vi "onListenForNewConnection.vi"(8 "error in (no error)":errorcluster, 9 "timeout (ms)":i32=1, 11 "Listener":refnum<class "WebsocketsConnection.lvclass">) -> (0 "error out":errorcluster, 1 "New connection":bool, 3 "New Connection":refnum<class "Connection.lvclass">)   [LabVIEW 2013, in "MQTT_Websockets.lvlib" / "WebsocketsConnection.lvclass"]
uses:
  WebsocketsConnection.lvclass
  MQTT_Connection/Connection/Connection.lvclass
  WebsocketsConnection.lvclass/WebsocketsConnection.ctl
  <vilib>/MediaMongrels Ltd/WebSockets/WebSockets/WebSocket Server/WebSocket Server.lvclass
  <vilib>/MediaMongrels Ltd/WebSockets/Sockets/VISA TCP Socket/VISA TCP.lvclass
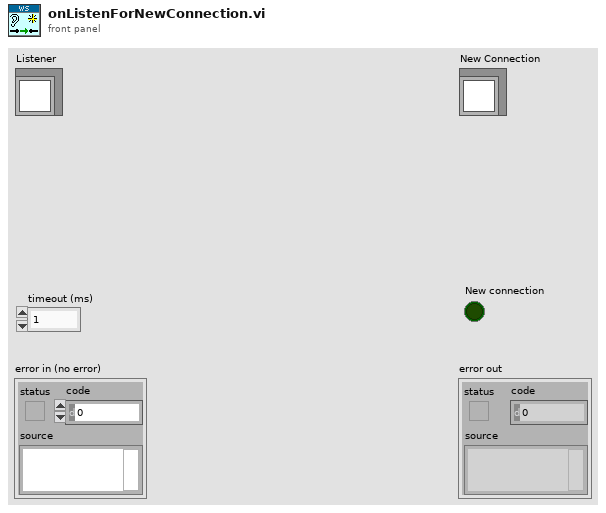
[diagram p1: front panel]
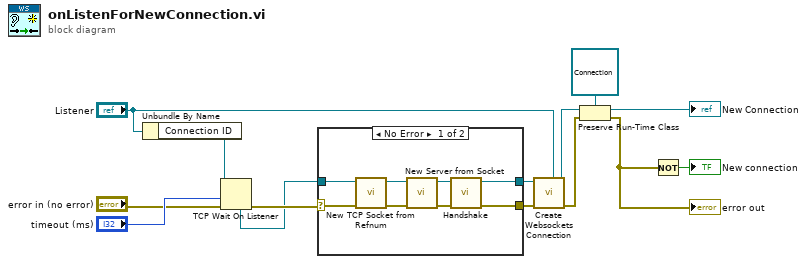
[diagram p0: block diagram]
diagram:
  n1 = Unbundle By Name("Listener") -> ("Connection ID"=w14:refnum<k5>)
  n2 = TCP Wait On Listener(8:"error in (no error)", 9:"timeout (ms)", 11:w14) -> (0:w8:errorcluster, 4:w1:refnum<k5>)  [unwired: 1 in, 3 out]
  n3 = case shown="No Error" w8 {
    selector: w8 -> [w16 w23]
    tunnel: [w20 _] -> w12
    tunnel: [w17 w23] -> w10
    tunnel: w1 -> [w15 _]
    frame No Error {
      n4 = call <vilib>:"New TCP Socket from Refnum.vi"("error in (no error)"=w16, "TCP Network Connection Refnum"=w15) -> ("error out"=w19:errorcluster, "VISA TCP out"=w22:refnum<class "VISA TCP.lvclass">)  [unwired: 8 in]
      n5 = call <vilib>:"New Server from Socket.vi"("error in (no error)"=w19, "Socket"=w22) -> ("error out"=w18:errorcluster, "WebSocket Server out"=w21:refnum<class "WebSocket Server.lvclass">)  [unwired: 8 in]
      n6 = call-dynamic "Handshake.vi"("error in (no error)"=w18, "WebSocket Connection in"=w21) -> ("error out"=w17:errorcluster, "WebSocket Connection out"=w20:refnum<class "WebSocket Server.lvclass">)  [unwired: 8 in]
    }
    frame Error {
    }
  }
  n7 = call "Create Websockets Connection.vi"("WSConnection in"="Listener", "error in (no error)"=w10, "WebSocket"=w12) -> ("error out"=w3:errorcluster, "WSConnection"=w6:refnum<class "WebsocketsConnection.lvclass">)  [unwired: 7 in]
  n8 = Preserve Run-Time Class(object in=w6, error in=w3, 2:refnum<class "Connection.lvclass"> refnum ("New Connection")) -> (object out=→"New Connection":refnum<class "Connection.lvclass">, error out=w2:errorcluster)
  "error out" <- w2
  n9 = Not(x=w2) -> (.not. x?=→"New connection":bool)
